vi "Junk1.vi"(10 "Numeric #2":dbl, 11 "Numeric #1":dbl) -> (3 "Numeric":dbl)   [LabVIEW 2018]
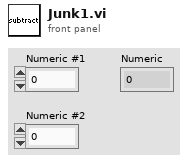
[diagram p1: front panel]
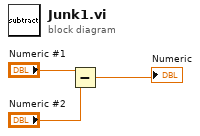
[diagram p0: block diagram]
diagram:
  n1 = Subtract(x="Numeric #1", y="Numeric #2") -> (x-y=→"Numeric":dbl)
